vi "TestCombine.vi"() -> ()   [LabVIEW 2016]
uses:
  <vilib>/Platform/TimedLoop/XDataNode/wakeup.ctl
  <vilib>/Platform/TimedLoop/XDataNode/XDNodeRunTimeDep.lvlib
  <vilib>/Platform/TimedLoop/XDataNode/nitl_modes.ctl
  <vilib>/Platform/TimedLoop/XDataNode/timing_clust.ctl
  <vilib>/Platform/TimedLoop/XDataNode/XDataNode.xnode
  <vilib>/robotics/Steering/Steering Frame/NI_Robotics_Steering Frame.lvclass
  <vilib>/myRIO/Instrument Drivers/Utilities/Utilities.lvlib
  <vilib>/robotics/Steering/Steering Frame/Apply Steering Frame Velocity to Wheels.vi
  <vilib>/robotics/Steering/Steering Frame/Get Steering Frame Velocity from Motors.vi
  <vilib>/robotics/Steering/Differential Steering Frame/NI_Robotics_Differential Steering Frame.lvclass
  C:/Program Files (x86)/National Instruments/LabVIEW 2016/vi.lib/robotics/Steering/Special Steering Frame/NI_Robotics_Special Steering Frame.lvclass
  C:/Program Files (x86)/National Instruments/LabVIEW 2016/vi.lib/robotics/Steering/Steering Frame/NI_Robotics_Steering Frame.lvclass
  <vilib>/robotics/Steering/Wheel/Rotation Direction.ctl
  <vilib>/robotics/Steering/Wheel/NI_Robotics_Wheel.lvclass
  <vilib>/robotics/Steering/Wheel/Wheel Parameters.ctl
  MotorControl/Configurations.ctl
panel:
  out "Obs_angle 2":dbl
  in  "Reset":bool
  in  "PID gains":T1
  out "element":cluster{"X":sgl, "Y":sgl, "theta":dbl}
  out "Waveform Chart 2":cluster{"theta":dbl, "Goal Heading":sgl}(graph)
  out "estimated steering frame posture":dbl[](array[numeric])
  out "estimated steering frame velocity":dbl[](array[numeric])
  out "appended array":dbl[](array[numeric])
  in  "Auto?":bool
  out "Frame Velocity Control":dbl[](array[numeric])
  out "Robot Position":cluster{dbl[], dbl[]}(graph)
  out "Goal list":cluster{"X":sgl, "Y":sgl, "theta":dbl}[](array[cluster])=[{"X"=3.0, "Y"=3.0, "theta"=0.0}, {"X"=5.0, "Y"=0.0, "theta"=0.0}]
  out "Obs_angle":dbl
  out "XY Graph":cluster{dbl[], dbl[]}[](graph)
  in  "Robot Configuration":T2={"wheel parameters"={"wheel radius"=0.05, "gear ratio"=1.0, "forward rotation direction"=0}, "wheel separation"=0.22, "Encoder Pulse Per Rev"=1920.0} {"wheel parameters"."forward rotation direction" items=["Clockwise", "Counterclockwise"]}
  out "Wheel Velocity":T5
  in  "steering frame velocity":dbl[](array[numeric])=[0.0, 0.0, 0.0]
  out "Waveform Chart":T6(graph)
  in  "stop":bool
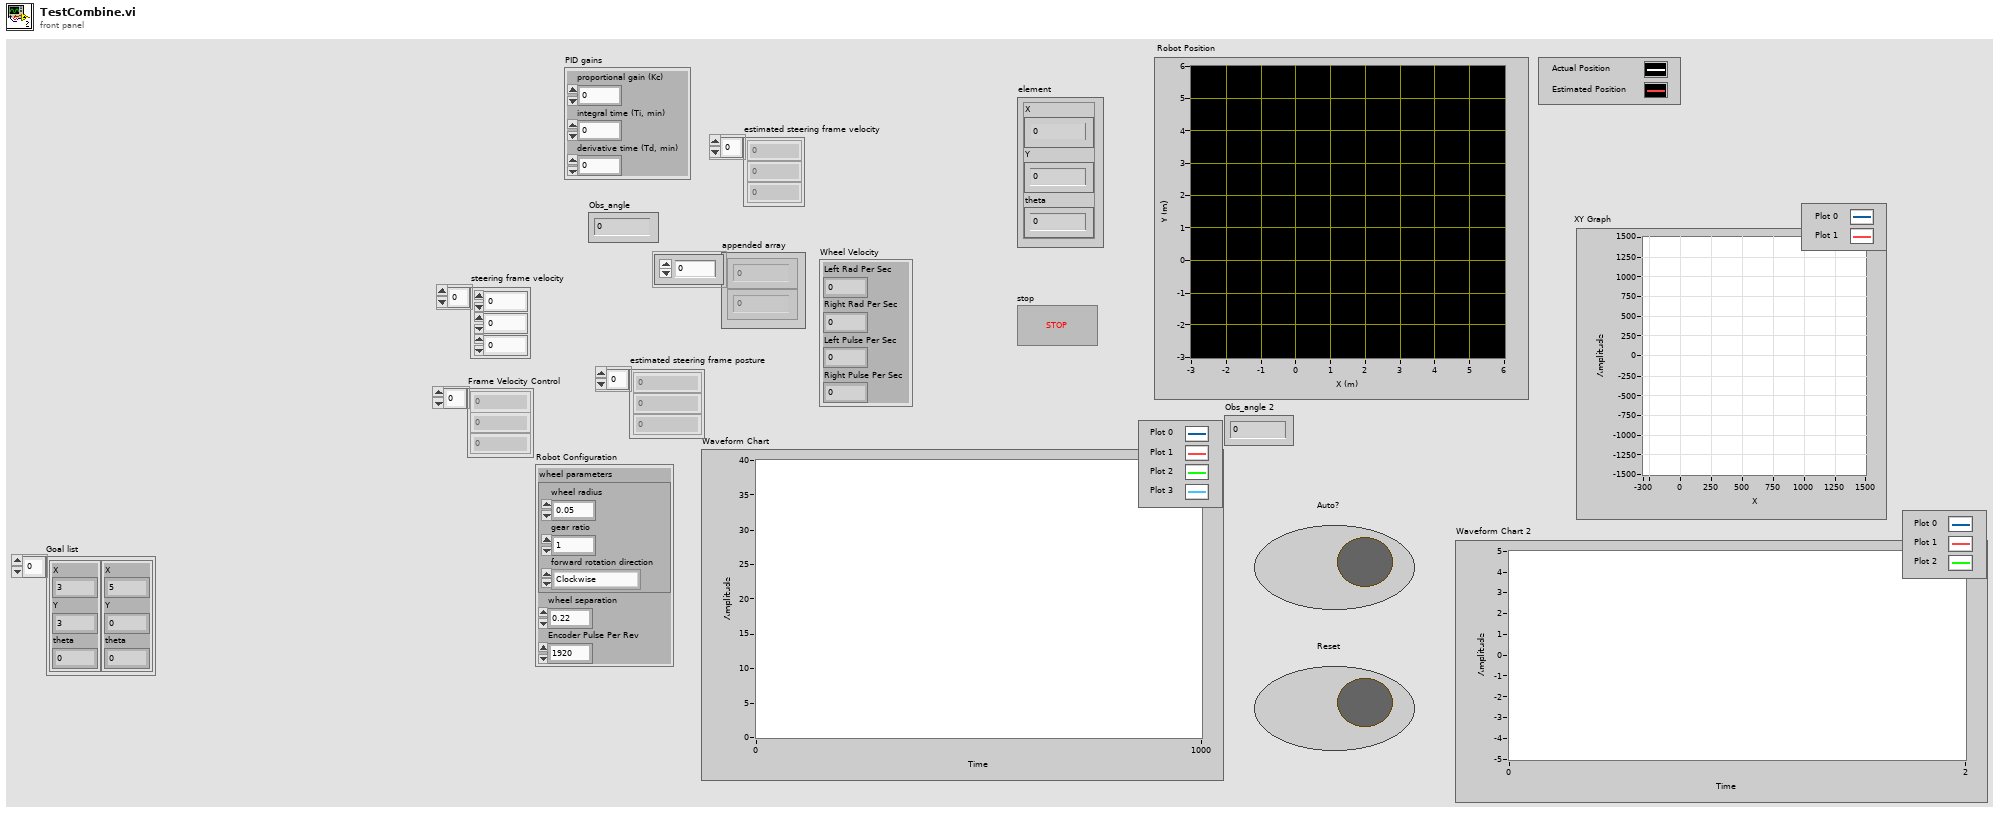
[diagram p1: front panel]
types:
  T1 = cluster{"proportional gain (Kc)":dbl, "integral time (Ti, min)":dbl, "derivative time (Td, min)":dbl}
  T2 = typedef "Configurations.ctl" = cluster{"wheel parameters":T3, "wheel separation":dbl, "Encoder Pulse Per Rev":dbl}
  T3 = typedef "NI_Robotics_Wheel.lvclass/Wheel Parameters.ctl" = cluster{"wheel radius":dbl, "gear ratio":dbl, "forward rotation direction":T4}
  T4 = typedef "NI_Robotics_Wheel.lvclass/Rotation Direction.ctl" = u16
  T5 = cluster{"Left Rad Per Sec":dbl, "Right Rad Per Sec":dbl, "Left Pulse Per Sec":dbl, "Right Pulse Per Sec":dbl}
  T6 = cluster{"forward angular velocity":dbl, dbl, "forward angular velocity":dbl, "Right Rad Per Sec":dbl}
  T7 = typedef "MotorObject.ctl" = cluster{"PWM Motor Left":T8, "PWM Motor Right":T8, "DIR Motor Left":T15, "Encoder Motor Left":T18, "Encoder Motor Right":T18, "DIR Motor Right":T15, "Left DIR Forward":bool}
  T8 = typedef "PWM.lvlib/PWM Reference.ctl" = cluster{"myRIO Reference":T9, "PWM Channels Enum":T13, "PWM Configuration":T14}
  T9 = typedef "myRIO Generic Hardware Reference.ctl" = cluster{"myRIO Model":T10, "myRIO Hardware Reference":T11}
  T10 = typedef "Hardware Version Enum.ctl" = enum16{"Unknown", "myRIO-1900", "myRIO-1950", "roboRIO", "NI ELVIS RIO CM"}
  T11 = typedef "myRIO v1.0 Reference.ctl" = cluster{"Generic FPGA Reference":T12, "Allow multiple opens":bool}
  T12 = typedef "Generic FPGA Reference.ctl" = refnum<k20>
  T13 = typedef "PWM Channels Enum.ctl" = enum16{"Not Connected", "C/PWM0", "C/PWM1", "A/PWM0", "A/PWM1", "A/PWM2", "B/PWM0", "B/PWM1", "B/PWM2", "PWM/PWM0", "PWM/PWM1", "PWM/PWM2", "PWM/PWM3", "PWM/PWM4", "PWM/PWM5", "PWM/PWM6", "PWM/PWM7", "PWM/PWM8", "PWM/PWM9"}
  T14 = typedef "PWM.lvlib/PWM Configuration.ctl" = cluster{"Frequency":dbl, "Duty Cycle":dbl}
  T15 = typedef "DIO.lvlib/DIO Reference.ctl" = cluster{"myRIO Reference":T9, "DIO Channels List":T16}
  T16 = typedef "DIO Channels List.ctl" = T17[]
  T17 = typedef "DIO Channels Enum.ctl" = enum16{"Not Connected", "C/DIO0", "C/DIO1", "C/DIO2", "C/DIO3", "C/DIO4", "C/DIO5", "C/DIO6", "C/DIO7", "A/DIO0", "A/DIO1", "A/DIO2", "A/DIO3", "A/DIO4", "A/DIO5", "A/DIO6", "A/DIO7", "A/DIO8", "A/DIO9", "A/DIO10", "A/DIO11", "A/DIO12", "A/DIO13", "A/DIO14", "A/DIO15", "B/DIO0", "B/DIO1", "B/DIO2", "B/DIO3", "B/DIO4", "B/DIO5", "B/DIO6", "B/DIO7", "B/DIO8", "B/DIO9", "B/DIO10", "B/DIO11", "B/DIO12", "B/DIO13", "B/DIO14", "B/DIO15", "LED0", "LED1", "LED2", "LED3", "Button0", "DIO/DIO0", "DIO/DIO1", "DIO/DIO2", "DIO/DIO3", "DIO/DIO4", "DIO/DIO5", "DIO/DIO6", "DIO/DIO7", "DIO/DIO8", "DIO/DIO9", "SPI/CS0", "SPI/CS1", "SPI/CS2", "SPI/CS3", "LED RADIO (Green)", "LED RADIO (Red)", "LED COMM (Green)", "LED COMM (Red)", "LED MODE (Green)", "LED MODE (Red)"}
  T18 = typedef "Encoder.lvlib/Encoder Reference.ctl" = cluster{"myRIO Reference":T9, "Encoder Channels Enum":T19}
  T19 = typedef "Encoder Channels Enum.ctl" = enum16{"Not Connected", "C/ENC0", "C/ENC1", "A/ENC", "B/ENC", "DIO/ENC0", "DIO/ENC1", "DIO/ENC2", "DIO/ENC3", "DIO/ENC4"}
  T20 = typedef "Measurement Parameters.ctl" = cluster{"Start Step":u32, "End Step":u32, "Cluster Count":u32, "Scan Interval":u32, "Number of Scans":u32, "Measurement Type":T21}
  T21 = typedef "Measurement Type.ctl" = enum16{"MS"}
  T22 = typedef "XDNodeRunTimeDep.lvlib/timing_clust.ctl" = cluster{"Expected End [f-1]":u64, "Actual End [f-1]":u64, "Finished Late? [f-1]":bool, "Expected End [i-1]":u64, "Actual End [i-1]":u64, "Finished Late? [i-1]":bool, "Expected Start [i]":u64, "Actual Start [i]":u64, "Expected Start [f]":u64, "Actual Start [f]":u64, "Source Name":string, "Structure Name":string, "Period":i64, "Deadline":i64, "Offset":i64, "Start":i64, "Priority":i32, "Timeout":i32, "Mode":T23, "Wakeup Reason":T24, "Error":errorcluster, "Source Type":string, "Secondary Source Type":string, "Global End Time":u64, "Global Start Time":u64, "Frame Duration":u64, "Iteration Duration":u64, "Assigned CPU":i32, "I/O Scan Engine Mode":u32}
  T23 = typedef "XDNodeRunTimeDep.lvlib/nitl_modes.ctl" = enum32{"No Change", "Process missed periods, maintain original phase", "Discard missed periods, maintain original phase", "Process missed periods, ignore original phase", "Discard missed periods, ignore original phase"}
  T24 = typedef "XDNodeRunTimeDep.lvlib/wakeup.ctl" = enum32{"Normal", "Aborted", "Asynchronous wakeup", "Timing source error", "Timed loop error", "Timeout"}
  T25 = cluster{"Angle to Goal":dbl, "Distance to Goal":sgl, "Goal Heading":sgl}
  T26 = typedef "NI_Robotics_Wheel.lvclass/Wheel State.ctl" = cluster{"wheel name":string, "forward angular velocity":dbl, "caster angular velocity":dbl, "caster wheel angle (rad)":dbl, "steering angle (rad)":dbl}
  T27 = cluster{"x_norm":dbl, "y_norm":dbl, "x LiDAR":dbl[], "y LiDAR":dbl[]}
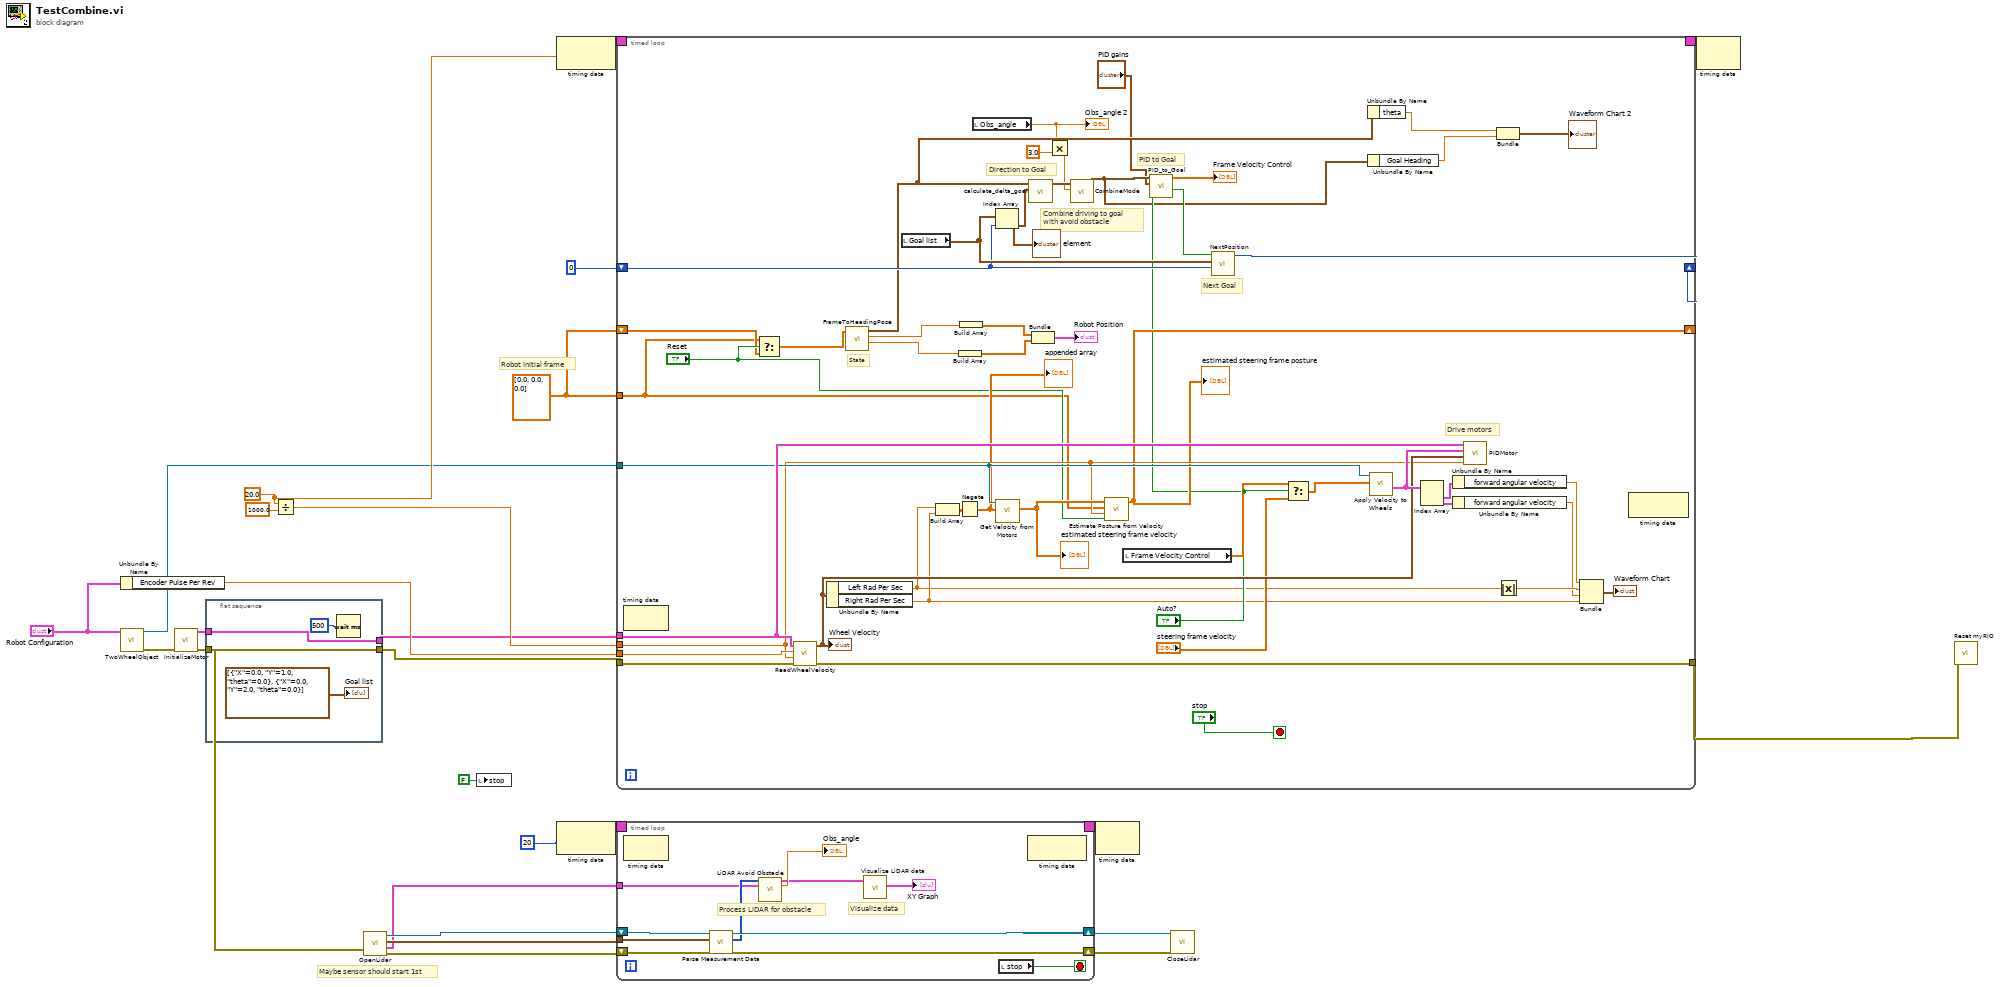
[diagram p0: block diagram]
diagram:
  w3 = dbl[] [0.0, 0.0, 0.0] ("initial posture")
  w24 = 20.0 ("Period")
  # "Robot initial frame"
  # "Maybe sensor should start 1st"
  n1 = Unbundle By Name("Robot Configuration") -> ("Encoder Pulse Per Rev"=w21:dbl)
  n2 = call "TwoWheelObject.vi"("Robot Configuration"="Robot Configuration") -> ("error out"=w6:errorcluster, "differential steering frame out"=w2:refnum<class "NI_Robotics_Differential Steering Frame.lvclass">)  [unwired: 9 in]
  n3 = call "InitializeMotor.vi"("error in"=w6) -> ("error out"=w18:errorcluster, "Motor Ref"=w16:T7)  [unwired: 9 in]
  n4 = flat-sequence {
    tunnel: w18 -> [w30]
    tunnel: [w30] -> w17
    tunnel: w16 -> [w28]
    tunnel: [w28] -> w15
    frame #0 {
      n5 = Wait (ms)(milliseconds to wait=u32 500) -> ()  [unwired: 1 out]
      "Goal list" <- cluster{"X":sgl, "Y":sgl, "theta":dbl}[] [{"X"=0.0, "Y"=1.0, "theta"=0.0}, {"X"=0.0, "Y"=2.0, "theta"=0.0}]
    }
  }
  n6 = Divide(x=w24, y=1000.0) -> (x/y=w22:dbl)
  n7 = call "OpenLidar.vi"("error in (no error)"=w6) -> ("error out"=w13:errorcluster, "Params Out"=w4:cluster{"angle":dbl[], "id":i32[], "kk":dbl[]}, "Measurement Parameters"=w10:T20, "VISA Refnum out"=w14:refnum<visa-resource-name>)  [unwired: 7 in]
  n8 = local write "stop"(FALSE ("stop")) -> ()
  n9 = node-c288(w24) -> (w26:T22)
  n10 = node-c288(i64 20 ("Period")) -> (w9:T22)
  n11 = timed-loop {
    timing: w26 -> [_]
    timing-out: [_] -> w25
    tunnel: w17 -> [w79]
    tunnel: w15 -> [w70]
    tunnel: w22 -> [w65]
    tunnel: w21 -> [w80]
    tunnel: [w78] -> w20
    tunnel: w2 -> [w67]
    tunnel: w3 -> [w38]
    shift-right: [w64] -> _
    shift-left: w3 -> [w39]
    shift-right: [w55] -> _
    shift-left: 0 -> [w53]
    stop <- "stop" stop-if-true
    # "Drive motors"
    # "Next Goal"
    # "Combine driving to goal \nwith avoid obstacle"
    # "PID to Goal"
    # "Direction to Goal"
    # "State"
    n12 = node-c288() -> ()  [unwired: 1 in, 1 out]
    n13 = Select(t=w38, s="Reset", f=w39) -> (s? t:f=w37:dbl[])
    n14 = call "ReadWheelVelocity.vi"("error in"=w79, "dt"=w65, "Encoder Pulse Per Rev"=w80, "Motor Ref"=w70) -> ("error out"=w78:errorcluster, "Wheel Velocity"=w68:T5)  [unwired: 6 in]
    "Wheel Velocity" <- w68
    n15 = Unbundle By Name(w68) -> ("Left Rad Per Sec"=w46:dbl, "Right Rad Per Sec"=w47:dbl)
    n16 = call "FrameToHeadingPose.vi"("Posture In"=w37) -> ("y"=w59:dbl, "x"=w60:dbl, "Heading Frame"=w44:cluster{"X":sgl, "Y":sgl, "theta":dbl})  [unwired: 8 in]
    n17 = local read "Goal list"() -> (w56:cluster{"X":sgl, "Y":sgl, "theta":dbl}[])
    n18 = Build Array(w46, w47) -> (w48:dbl[])
    n19 = Build Array(w59) -> (w62:dbl[])
    n20 = Negate(x=w48) -> (-x=w45:dbl[])
    "appended array" <- w45
    n21 = Build Array(w60) -> (w63:dbl[])
    n22 = local read "Obs_angle"() -> (w33:dbl)
    "Obs_angle 2" <- w33
    n23 = Index Array(array=w56, index=w53) -> (element=w58:cluster{"X":sgl, "Y":sgl, "theta":dbl})
    "element" <- w58
    n24 = call-poly <vilib>:"Get Velocity from Motors.vi"("ccw motor velocity states"=w45, "steering frame in"=w67) -> ("estimated steering frame velocity"=w66:dbl[])  [unwired: 7 in, 2 out]
    "estimated steering frame velocity" <- w66
    n25 = call "calculate_delta_goal.vi"("Goal State"=w58, "Robot State"=w44) -> ("Output to Goal"=w43:T25)  [unwired: 9 in]
    n26 = Bundle(w63, w62) -> (→"Robot Position":cluster{dbl[], dbl[]})  [unwired: 1 in]
    n27 = Multiply(x=w33, y=3.0) -> (x*y=w32:dbl)
    n28 = call "CombineMode.vi"("Obstacle Angle"=w32, "Output to Goal in"=w43) -> ("Output to Goal out"=w35:T25)  [unwired: 9 in]
    n29 = call "Estimate Posture from Velocity.vi"("initialize"="Reset", "dt (s)"=w65, "initial posture"=w38, "estimated steering frame velocity"=w66) -> ("estimated steering frame posture"=w64:dbl[])  [unwired: 7 in]
    "estimated steering frame posture" <- w64
    n30 = local read "Frame Velocity Control"() -> (w50:dbl[])
    n31 = call "PID_to_Goal.vi"("Boolean"="Auto?", "PID gains"="PID gains", "Direction to Goal"=w35) -> ("Goal Arrive?"=w54:bool, "Frame Velocity"=→"Frame Velocity Control":dbl[])  [unwired: 6 in, 1 out]
    n32 = call "NextPosition.vi"("Numeric Control in"=w53, "Goal list"=w56, "Goal Arrive?"=w54) -> ("Numeric Control out"=w55:i32)  [unwired: 8 in]
    n33 = Select(t=w50, s="Auto?", f="steering frame velocity") -> (s? t:f=w51:dbl[])
    n34 = Unbundle By Name(w35) -> ("Goal Heading"=w41:sgl)
    n35 = Unbundle By Name(w44) -> ("theta"=w42:dbl)
    n36 = call-poly <vilib>:"Apply Velocity to Wheels.vi"("steering frame velocity"=w51, "steering frame in"=w67) -> ("calculated wheel states"=w69:T26[])  [unwired: 6 in, 3 out]
    n37 = Index Array(array=w69) -> (element #1=w77:T26, element #2=w76:T26)  [unwired: 2 in]
    n38 = Unbundle By Name(w77) -> ("forward angular velocity"=w75:dbl)
    n39 = Unbundle By Name(w76) -> ("forward angular velocity"=w72:dbl)
    n40 = call "PIDMotor.vi"("Motor Object"=w70, "calculated wheel states"=w69, "Wheel Velocity"=w68, "dt"=w65) -> ()  [unwired: 7 in]
    n41 = Bundle("theta"=w42, "Goal Heading"=w41) -> (→"Waveform Chart 2":cluster{"theta":dbl, "Goal Heading":sgl})  [unwired: 1 in]
    n42 = Absolute Value(x=w46) -> (abs(x)=w73:dbl)
    n43 = Bundle("forward angular velocity"=w75, w73, "forward angular velocity"=w72, "Right Rad Per Sec"=w47) -> (→"Waveform Chart":T6)  [unwired: 1 in]
    n44 = node-c288() -> ()  [unwired: 1 in, 1 out]
  }
  n45 = timed-loop {
    tunnel: w10 -> [w92]
    shift-right: [w88] -> w12
    shift-left: w14 -> [w91]
    shift-right: [w89] -> w11
    shift-left: w13 -> [w90]
    timing: w9 -> [_]
    timing-out: [_] -> w8
    tunnel: w4 -> [w85]
    stop <- w86 stop-if-true
    # "Process LiDAR for obstacle"
    # "Visualize data"
    n46 = node-c288() -> ()  [unwired: 1 in, 1 out]
    n47 = call "Parse Measurement Data.vi"("error in (no error)"=w90, "Measurement Parameters"=w92, "VISA Refnum in"=w91) -> ("error out"=w89:errorcluster, "Measurement Data"=w87:i32[], "VISA Refnum out"=w88:refnum<visa-resource-name>)  [unwired: 6 in]
    n48 = call "LiDAR Avoid Obstacle.vi"("Measurement Data"=w87, "Input Params"=w85) -> ("Output data"=w83:T27, "Obs_angle"=→"Obs_angle":dbl)  [unwired: 12 in]
    n49 = call "Visualize LiDAR data.vi"("Input LiDAR"=w83) -> ("Array"=→"XY Graph":cluster{"x LiDAR":dbl[], "y LiDAR":dbl[]}[])  [unwired: 10 in]
    n50 = local read "stop"() -> (w86:bool)
    n51 = node-c288() -> ()  [unwired: 1 in, 1 out]
  }
  n52 = node-c288(w8) -> ()  [unwired: 1 out]
  n53 = call "CloseLidar.vi"("error in (no error)"=w11, "VISA Refnum in"=w12) -> ()  [unwired: 10 in]
  n54 = node-c288(w25) -> ()  [unwired: 1 out]
  n55 = call <vilib>:"Reset myRIO.vi"("error in (no error)"=w20) -> ()  [unwired: 10 in, 1 out]
